vi "SET_DEVICE_OUTPUT_VBAT_TO_GLOBAL.vi"(6 "VBAT":dbl, 7 "OUTPUT":bool, 10 "DEVICE":string, 11 "USB_DEV":string) -> (2 "JSON string response TO USB DEV":string, 3 "Dev?":bool)   [LabVIEW 2015]
uses:
  Share Data/uPower_kit.ctl
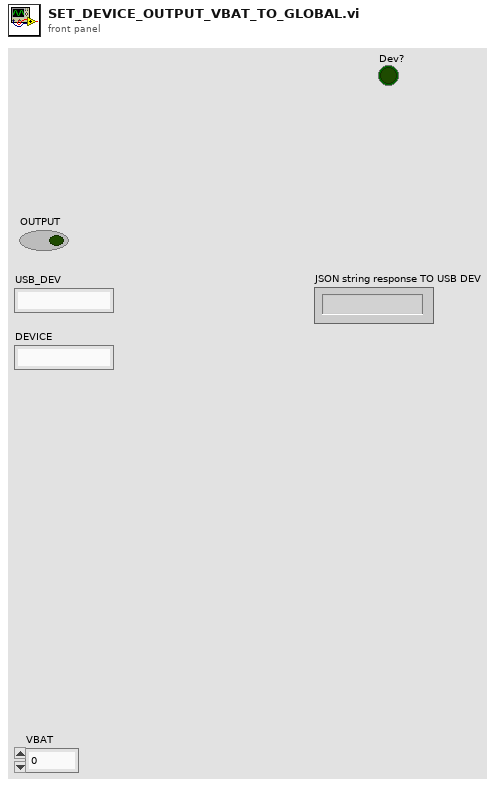
[diagram p1: front panel]
types:
  T1 = typedef "uPower_kit.ctl" = cluster{"DEV":string, "BUSY":bool, "VBAT":dbl, "OUTPUT":bool, "LAST_RESULT":dbl, "DURATION":u16, "TRIGGER":bool, "RANGE":string, "Vsource":dbl}
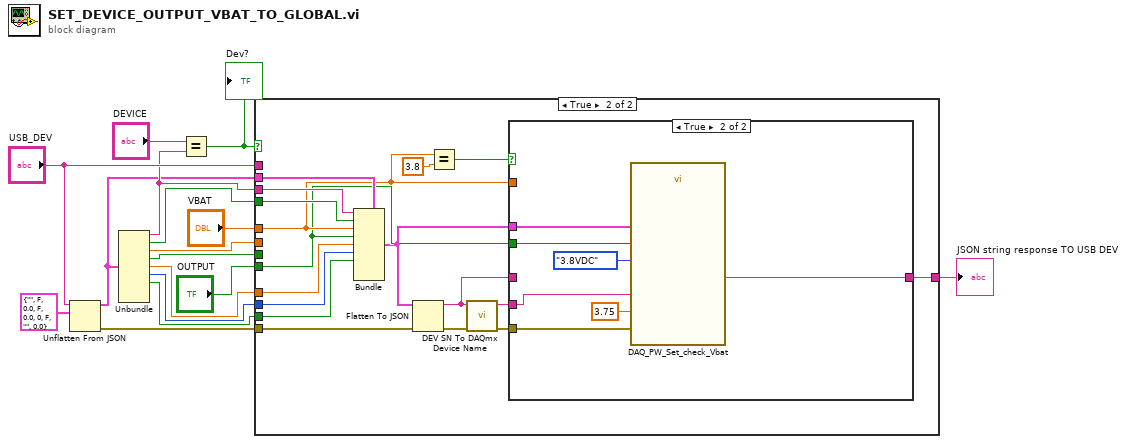
[diagram p0: block diagram]
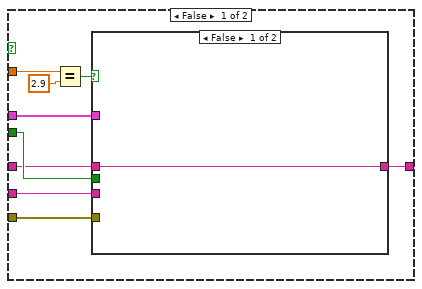
[diagram p3: hidden frame]
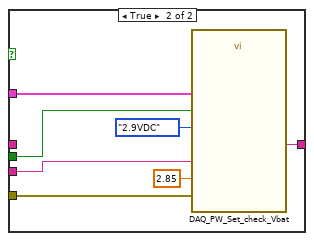
[diagram p4: hidden frame]
diagram:
  n1 = Unflatten From JSON(JSON string="USB_DEV", type and defaults=T1 {"DEV"="", "BUSY"=FALSE, "VBAT"=0.0, "OUTPUT"=FALSE, "LAST_RESULT"=0.0, "DURATION"=0, "TRIGGER"=FALSE, "RANGE"="", "Vsource"=0.0} ("DEV_BUSY")) -> (value=w6:T1, error out=w1:errorcluster)  [unwired: 5 in]
  n2 = Unbundle(w6) -> ("DEV"=w9:string, "BUSY"=w10:bool, "VBAT"=w11:dbl, "OUTPUT"=w12:bool, "LAST_RESULT"=w13:dbl, "DURATION"=w3:u16, "TRIGGER"=w2:bool)  [unwired: 2 out]
  n3 = Equal?(x="DEVICE", y=w9) -> (x = y?=w8:bool)
  "Dev?" <- w8
  n4 = case shown="True" w8 {
    tunnel: w6 -> [_ w34]
    tunnel: w9 -> [_ w33]
    tunnel: w10 -> [_ w32]
    tunnel: w11 -> [_ _]
    tunnel: w12 -> [_ _]
    tunnel: w13 -> [_ w31]
    tunnel: "VBAT" -> [_ w26]
    tunnel: "OUTPUT" -> [_ w21]
    tunnel: [w17 w18] -> w4
    tunnel: "USB_DEV" -> [w17 _]
    tunnel: w3 -> [_ w30]
    tunnel: w2 -> [_ w29]
    tunnel: w1 -> [_ w22]
    frame False {
    }
    frame True {
      n5 = Bundle(cluster=w34, "DEV"=w33, "BUSY"=w32, "VBAT"=w26, "OUTPUT"=w21, "LAST_RESULT"=w31, "DURATION"=w30, "TRIGGER"=w29) -> (w20:T1)  [unwired: 2 in]
      n6 = Flatten To JSON(anything=w20, error in (no error)=w22) -> (JSON string=w19:string, 11:w23:errorcluster)  [unwired: 1 in]
      n7 = Equal?(x=w26, y=3.8) -> (x = y?=w27:bool)
      n8 = call "DEV SN To DAQmx Device Name.vi"("error in (no error)"=w23, "USN_DEV (JSON)"=w19) -> ("error out"=w25:errorcluster, "DAQmx Device Name"=w24:tag)  [unwired: 8 in]
      n9 = case shown="True" w27 {
        tunnel: w26 -> [w43 _]
        tunnel: w25 -> [w40 w57]
        tunnel: w24 -> [w39 w52]
        tunnel: w21 -> [w38 w56]
        tunnel: w20 -> [w37 w55]
        tunnel: w19 -> [w36 _]
        tunnel: [w35 w53] -> w18
        frame False {
          n10 = Equal?(x=w43, y=2.9) -> (x = y?=w41:bool)
          n11 = case shown="False" w41 {
            tunnel: w40 -> [_ w46]
            tunnel: w39 -> [_ w47]
            tunnel: w38 -> [_ w48]
            tunnel: w37 -> [_ w49]
            tunnel: [w44 w45] -> w35
            tunnel: w36 -> [w44 _]
            frame False {
            }
            frame True {
              n12 = call "DAQ_PW_Set_check_Vbat.vi"("Vbat_set"=2.85 ("y"), "DEV_BUSY"=w49, "error in (no error)"=w46, "DUT Voltage Selector"=enum16{"3.8VDC", "2.9VDC", "3.7VDC", "4.0VDC"}."2.9VDC", "DAQmx Device Name"=w47, "OUTPUT"=w48) -> ("JSON string"=w45:string)  [unwired: 5 in]
            }
          }
        }
        frame True {
          n13 = call "DAQ_PW_Set_check_Vbat.vi"("Vbat_set"=3.75 ("y"), "DEV_BUSY"=w55, "error in (no error)"=w57, "DUT Voltage Selector"=enum16{"3.8VDC", "2.9VDC", "3.7VDC", "4.0VDC"}."3.8VDC", "DAQmx Device Name"=w52, "OUTPUT"=w56) -> ("JSON string"=w53:string)  [unwired: 5 in]
        }
      }
    }
  }
  "JSON string response TO USB DEV" <- w4
